vi "Override To Nominal State.vi"(11 "TEMPLATE Event in":refnum<class "TEMPLATE Event.lvclass">) -> (3 "TEMPLATE Event out":refnum<class "TEMPLATE Event.lvclass">)   [LabVIEW 2021, in "_Template.lvlib" / "Templates.lvlib" / "TEM Event.lvlib" / "TEMPLATE Event.lvclass"]
uses:
  TEMPLATE Event.lvclass
  TEMPLATE Event.lvclass/TEMPLATE Event.ctl
  <vilib>/Nathan Davis/jettl/jettl/Event/Event.lvclass
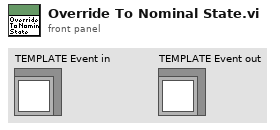
[diagram p1: front panel]
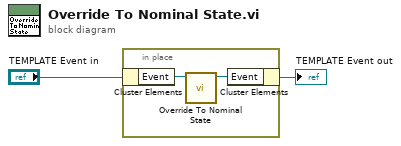
[diagram p0: block diagram]
diagram:
  n1 = in-place {
    n2 = in-place-cluster #1("TEMPLATE Event in") -> ("Event"=w4:refnum<class "Event.lvclass">)
    n3 = call-dynamic "Override To Nominal State.vi"("jettl in"=w4) -> ("jettl out"=w3:refnum<class "Event.lvclass">)  [unwired: 10 in]
    n4 = in-place-cluster #1("Event"=w3) -> (→"TEMPLATE Event out":refnum<class "TEMPLATE Event.lvclass">)
  }
